vi "Simple Splash Screen 2012 NIVerified.vi"(7 "Start Splash Screen":bool, 8 "error in (no error)":errorcluster) -> (0 "error out":errorcluster)   [LabVIEW 2023]
panel:
  # "Overview: This example VI shows how to implement the splash screen in LabVIEW.\nRequirements: LabVIEW Base Development System 2012 (or compatible)\nInstructions:\n1.\tRun the program.\n2.\tObserve the splash screen."
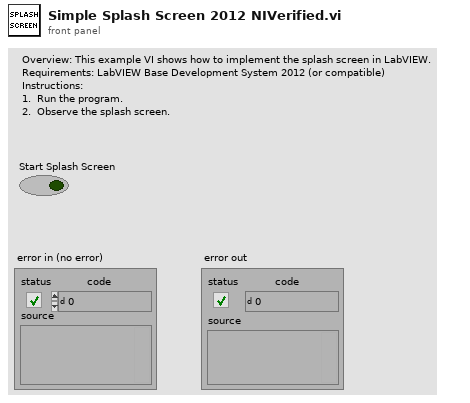
[diagram p1: front panel]
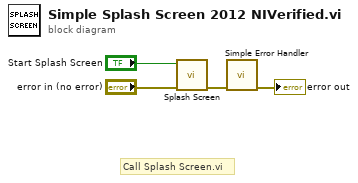
[diagram p0: block diagram]
diagram:
  # "Call Splash Screen.vi"
  n1 = call "Splash Screen.vi"("error in (no error)"="error in (no error)", "Start Splash Screen"="Start Splash Screen") -> ("error out"=w4:errorcluster)  [unwired: 9 in]
  n2 = call <vilib>:"Simple Error Handler.vi"("error in (no error)"=w4) -> ("error out"=→"error out":errorcluster)  [unwired: 4 in, 4 out]
